vi "Read Checked.vi"(8 "error in (no error)":errorcluster, 11 "MenuItem in":refnum<class "MGI_MenuItem.lvclass">) -> (0 "error out":errorcluster, 2 "Checked":bool, 3 "MenuItem out":refnum<class "MGI_MenuItem.lvclass">)   [LabVIEW 2016, in "MGI_MenuItem.lvclass"]
doc: "Authored by Derek E. Trepanier\nsupport@mooregoodideas.com\nwww.mooregoodideas.com\n\nCopyright (c) 2012, Moore Good Ideas, Inc.\n\nAll rights reserved.\n\nRedistribution and use in source and binary forms, with or without modification, are permitted provided that the following conditions are met:\n\n * Redistributions of source code must retain the above copyright notice, this list of conditions and the following disclaimer.\n * Redistributions in binary form must reproduce the above copyright notice, this list of conditions and the following disclaimer in the documentation and/or other materials provided with the distribution.\n * Neither the name of Moore Good Ideas, Inc. nor the names of its contributors may be used to endorse or promote products derived from this software without specific prior written permission.\n\nTHIS SOFTWARE IS PROVIDED BY THE COPYRIGHT HOLDERS AND CONTRIBUTORS \"AS IS\" AND ANY EXPRESS OR IMPLIED WARRANTIES, INCLUDING, BUT NOT LIMITED TO, THE IMPLIED WARRANTIES OF MERCHANTABILITY AND FITNESS FOR A PARTICULAR PURPOSE ARE DISCLAIMED. IN NO EVENT SHALL THE COPYRIGHT OWNER OR CONTRIBUTORS BE LIABLE FOR ANY DIRECT, INDIRECT, INCIDENTAL, SPECIAL, EXEMPLARY, OR CONSEQUENTIAL DAMAGES (INCLUDING, BUT NOT LIMITED TO, PROCUREMENT OF SUBSTITUTE GOODS OR SERVICES; LOSS OF USE, DATA, OR PROFITS; OR BUSINESS INTERRUPTION) HOWEVER CAUSED AND ON ANY THEORY OF LIABILITY, WHETHER IN CONTRACT, STRICT LIABILITY, OR TORT (INCLUDING NEGLIGENCE OR OTHERWISE) ARISING IN ANY WAY OUT OF THE USE OF THIS SOFTWARE, EVEN IF ADVISED OF THE POSSIBILITY OF SUCH DAMAGE."
uses:
  <userlib>/_MGI/Menu Building/MenuItem/MGI_MenuItem.lvclass
  <userlib>/_MGI/Menu Building/MenuItem/MGI_MenuItem.lvclass/MGI_MenuItem.ctl
  <userlib>/_MGI/Menu Building/MenuTypes/MGI_Menu.lvclass
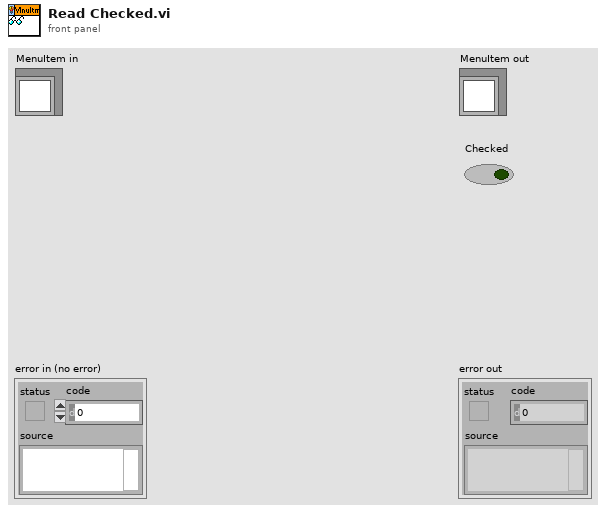
[diagram p1: front panel]
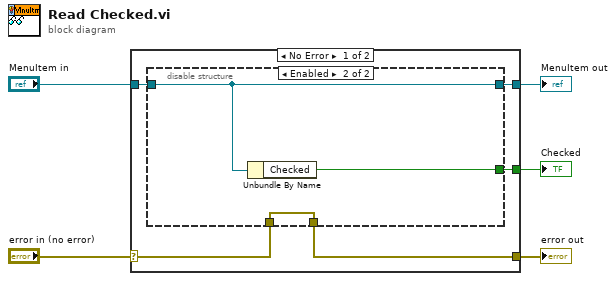
[diagram p0: block diagram]
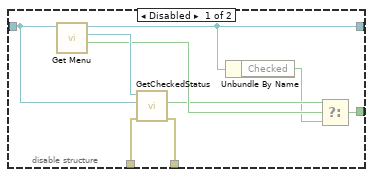
[diagram p2: hidden frame]
diagram:
  n1 = case shown="No Error" "error in (no error)" {
    selector: "error in (no error)" -> [w7 w23]
    tunnel: [w6 w23] -> w4
    tunnel: [w10 w24] -> w2
    tunnel: "MenuItem in" -> [w9 w24]
    tunnel: [w8 _] -> w1
    frame No Error {
      n2 = disable-structure shown="Enabled" {
        disable-tunnel: [w19 w22] -> w10
        disable-tunnel: w9 -> [w17 w22]
        disable-tunnel: [w16 w20] -> w8
        disable-tunnel: w7 -> [w12 w21]
        disable-tunnel: [w11 w21] -> w6
        frame Disabled {
          n3 = call <userlib>:"Get Menu.vi"("MenuItem in"=w17) -> ("Menu Valid"=w15:bool, "Menu"=w18:refnum<class "MGI_Menu.lvclass">, "MenuItem out"=w19:refnum<class "MGI_MenuItem.lvclass">)  [unwired: 7 in, 1 out]
          n4 = call-dynamic "GetCheckedStatus.vi"("error in (no error)"=w12, "MenuItem"=w17, "Menu in"=w18) -> ("error out"=w11:errorcluster, "Checked?"=w14:bool)  [unwired: 6 in, 1 out]
          n5 = Unbundle By Name(w19) -> ("Checked"=w13:bool)
          n6 = Select(t=w14, s=w15, f=w13) -> (s? t:f=w16:bool)
        }
        frame Enabled {
          n7 = Unbundle By Name(w22) -> ("Checked"=w20:bool)
        }
      }
    }
    frame Error {
    }
  }
  "error out" <- w4
  "MenuItem out" <- w2
  "Checked" <- w1
